vi "PCE-TestGUI.vi"() -> ()   [LabVIEW 2011]
panel:
  out "Actif":bool
  in  "DEC":dbl=3.0 min=3.0 max=1800.0 step=1.0
  in  "RA":dbl=30.0 min=3.0 max=1800.0 step=1.0
  in  "Offset":bool
  out "Data Cluster":T1={"HA"=0.882, "RA"=11305.911600000001, "DEC"=127486.3032, "Epoque"=2000.0, "Masse d'air"=1.015373, "Temps Sidéral"=11356.938, "Temps Universel"=65621.232, "Année"=2013.290212, "Focus"=5325.0, "Dome"=359.999912, "Rotateur"=-108.7074} {"Rotateur" format="%.2f"; "Dome" format="%.2f"; "Focus" format="%.2f"; "Année" format="%.2f"; "Temps Universel" format="%<%H:%M:%S%0u>t"; "Temps Sidéral" format="%<%H:%M:%S%0u>t"; "Masse d'air" format="%.2f"; "Epoque" format="%.2f"; "DEC" format="%<%H:%M:%S%0u>t"; "RA" format="%<%H:%M:%S%0u>t"; "HA" format="%<%H:%M:%S%0u>t"}
  in  "Info":bool
  in  "Quit":bool
  in  "Port":u16=8380
  in  "IP":string="132.204.61.80"
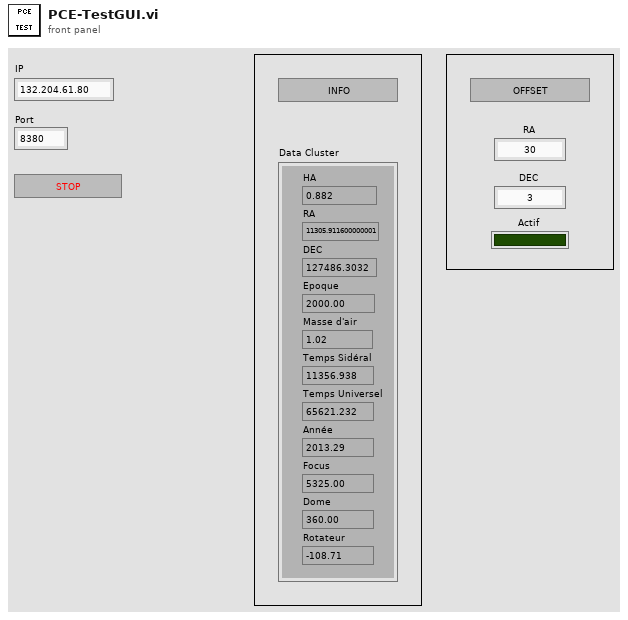
[diagram p1: front panel]
types:
  T1 = cluster{"HA":dbl, "RA":dbl, "DEC":dbl, "Epoque":dbl, "Masse d'air":dbl, "Temps Sidéral":dbl, "Temps Universel":dbl, "Année":dbl, "Focus":dbl, "Dome":dbl, "Rotateur":dbl}
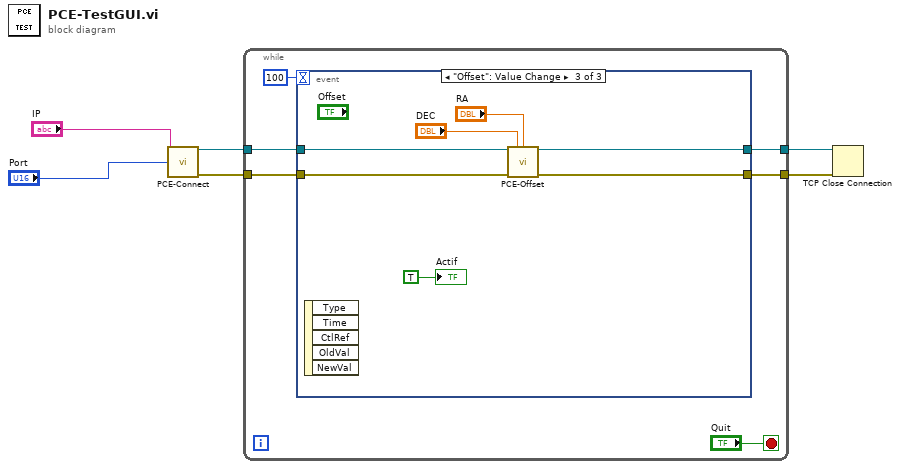
[diagram p0: block diagram]
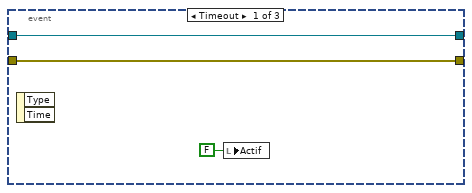
[diagram p2: hidden frame]
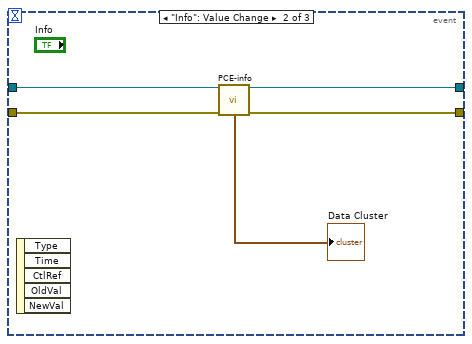
[diagram p3: hidden frame]
diagram:
  n1 = call "PCE-Connect.vi"("IP"="IP", "Port"="Port") -> ("connection ID"=w4:refnum<k5>, "error out"=w3:errorcluster)  [unwired: 12 in]
  n2 = while {
    tunnel: w4 -> [w10]
    tunnel: w3 -> [w9]
    tunnel: [w8] -> w2
    tunnel: [w7] -> w1
    stop <- "Quit" stop-if-true
    n3 = event shown="[2] \"Offset\": Value Change" {
      selector: _ -> [_ _ _]
      dyn-events: _ -> [_ _ _]
      timeout: 100 -> [_ _ _]
      tunnel: w10 -> [w15 w20 w27]
      tunnel: w9 -> [w14 w19 w22]
      tunnel: [w15 w18 w26] -> w8
      tunnel: [w14 w17 w25] -> w7
      event Timeout {
        n4 = event-data() -> ()  [unwired: 1 in, 2 out]
        n5 = local write "Actif"(FALSE ("Actif")) -> ()
      }
      event "Info": Value Change {
        n6 = event-data() -> ()  [unwired: 1 in, 5 out]
        n7 = call "PCE-info.vi"("connection ID"=w20, "error in"=w19) -> ("connection ID dup"=w18:refnum<k5>, "Data Cluster"=→"Data Cluster":T1, "error out"=w17:errorcluster)  [unwired: 11 in]
      }
      event "Offset": Value Change {
        n8 = event-data() -> ()  [unwired: 1 in, 5 out]
        n9 = call "PCE-Offset.vi"("connection ID"=w27, "DEC"="DEC", "RA"="RA", "error in"=w22) -> ("connection ID dup"=w26:refnum<k5>, "error out"=w25:errorcluster)  [unwired: 10 in]
        "Actif" <- TRUE ("Actif")
      }
    }
  }
  n10 = TCP Close Connection(connection ID=w2, error in (no error)=w1) -> ()  [unwired: 1 in, 2 out]
